vi "IMAQ-MWT (FPGA) without PA and Arduino Interface.vi"() -> ()   [LabVIEW 2015]
uses:
  <vilib>/eio/EIONode/EIONode.xnode
  <vilib>/rvi/eio/common/nirviEmuTemplateMethod_errors.vi
  <vilib>/Platform/TimedLoop/XDataNode/wakeup.ctl
  <vilib>/Platform/TimedLoop/XDataNode/XDNodeRunTimeDep.lvlib
  <vilib>/Platform/TimedLoop/XDataNode/nitl_modes.ctl
  <vilib>/Platform/TimedLoop/XDataNode/timing_clust.ctl
  <vilib>/Platform/TimedLoop/XDataNode/XDataNode.xnode
  Modules/Common/Controls (FPGA)/Pixel Bundle 40 Bytes.ctl
  <vilib>/rvi/DataTransferAndStorage/Container/XNode/niFpgaContainer.xnode
  <vilib>/rvi/FIFO/Fifo_Resource/nirvififoEmulationWrite.vi
  <vilib>/rvi/FIFO/Fifo_Resource/nirvififoEmulationRead.vi
  <vilib>/rvi/interface/RandomDataEmulation/nirviRandomDataFpgaReadWriteTemplate.vi
  Modules/CL Data to Pixels/8 Tap 8-Bit.vi
  Modules/CL Data to Pixels/10 Tap 8-Bit.vi
  Modules/Common/Controls (FPGA)/CL Configuration.ctl
  Modules/Common/Controls (FPGA)/CL Signal Mapping.ctl
  <vilib>/rvi/LocalResourceManager/LocalResourceManager.xnode
  <vilib>/rvi/DataTransferAndStorage/Container/Common/niFpgaContainerGetUniqueNameForEmu.vi
  <vilib>/rvi/DataTransferAndStorage/Container/Common/niFpgaContainerSetEmuInfo.vi
  <vilib>/rvi/eio/common/nirviEmuReportErrorAndStop.vi
  Modules/Common/Controls (FPGA)/Data to Arduino.ctl
  Modules/Common/Controls (FPGA)/Camera Tap Configuration.ctl
  Modules/Common/Controls (FPGA)/Run Mode.ctl
panel:
  in  "Baud Rate":u32=500000
  in  "N Spline Points":fxp<+,8,8>=31.0
  in  "Clock Cycles Limit":u32=10000
  in  "Pixel Intensity":cluster{"Low":u8, "High":u8}={"Low"=100, "High"=255}
  out "Frame Interval":u32=4294967295
  out "Frame #":u32
  out "DMA Timeout":bool
  in  "Mode":T1
  in  "Image Height":u16=3072
  in  "Image Width":u16=3072
  in  "Cancel Acq":bool
  in  "Acquire":bool
  out "Acq In Progress":bool
  in  "Tap Configuration":T2
  in  "Initialize":bool=TRUE
  out "Initialized":bool=TRUE
  # "IMAQ - MWT"
  # "Camera Link Configuration"
  # "Object Detection"
  # "Acquisition Settings"
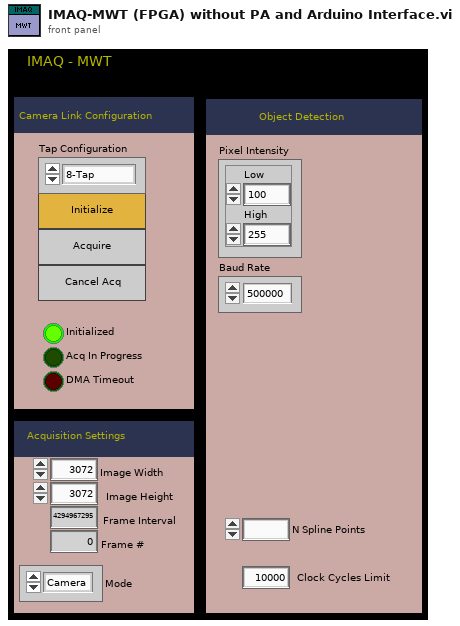
[diagram p1: front panel]
types:
  T1 = typedef "Run Mode.ctl" = enum16{"Camera", "Video (Raw)", "Video (DBDE)"}
  T2 = typedef "Camera Tap Configuration.ctl" = enum8{"8-Tap", "10-Tap"}
  T3 = typedef "CL Signal Mapping.ctl" = enum8{"Standard", "Basler 10-tap", "Vosskühler 10-tap"}
  T4 = typedef "CL Configuration.ctl" = enum8{"Base", "Medium", "Full"}
  T5 = typedef "XDNodeRunTimeDep.lvlib/timing_clust.ctl" = cluster{"Expected End [f-1]":u64, "Actual End [f-1]":u64, "Finished Late? [f-1]":bool, "Expected End [i-1]":u64, "Actual End [i-1]":u64, "Finished Late? [i-1]":bool, "Expected Start [i]":u64, "Actual Start [i]":u64, "Expected Start [f]":u64, "Actual Start [f]":u64, "Source Name":string, "Structure Name":string, "Period":i64, "Deadline":i64, "Offset":i64, "Start":i64, "Priority":i32, "Timeout":i32, "Mode":T6, "Wakeup Reason":T7, "Error":errorcluster, "Source Type":string, "Secondary Source Type":string, "Global End Time":u64, "Global Start Time":u64, "Frame Duration":u64, "Iteration Duration":u64, "Assigned CPU":i32, "I/O Scan Engine Mode":u32}
  T6 = typedef "XDNodeRunTimeDep.lvlib/nitl_modes.ctl" = enum32{"No Change", "Process missed periods, maintain original phase", "Discard missed periods, maintain original phase", "Process missed periods, ignore original phase", "Discard missed periods, ignore original phase"}
  T7 = typedef "XDNodeRunTimeDep.lvlib/wakeup.ctl" = enum32{"Normal", "Aborted", "Asynchronous wakeup", "Timing source error", "Timed loop error", "Timeout"}
  T8 = typedef "Pixel Bundle 40 Bytes.ctl" = cluster{"Pixel 1":u8, "Pixel 2":u8, "Pixel 3":u8, "Pixel 4":u8, "Pixel 5":u8, "Pixel 6":u8, "Pixel 7":u8, "Pixel 8":u8, "Pixel 9":u8, "Pixel 10":u8, "Pixel 11":u8, "Pixel 12":u8, "Pixel 13":u8, "Pixel 14":u8, "Pixel 15":u8, "Pixel 16":u8, "Pixel 17":u8, "Pixel 18":u8, "Pixel 19":u8, "Pixel 20":u8, "Pixel 21":u8, "Pixel 22":u8, "Pixel 23":u8, "Pixel 24":u8, "Pixel 25":u8, "Pixel 26":u8, "Pixel 27":u8, "Pixel 28":u8, "Pixel 29":u8, "Pixel 30":u8, "Pixel 31":u8, "Pixel 32":u8, "Pixel 33":u8, "Pixel 34":u8, "Pixel 35":u8, "Pixel 36":u8, "Pixel 37":u8, "Pixel 38":u8, "Pixel 39":u8, "Pixel 40":u8}
  T9 = cluster{"Enables Valid":bool, "Frame Valid":bool, "Line Valid":bool, "Data Valid":bool}
  T10 = cluster{"Pixel 0":u8, "Pixel 1":u8, "Pixel 2":u8, "Pixel 3":u8, "Pixel 4":u8, "Pixel 5":u8, "Pixel 6":u8, "Pixel 7":u8, "Pixel 8":u8, "Pixel 9":u8}
  T11 = cluster{"Pixel 0":u8, "Pixel 1":u8, "Pixel 2":u8, "Pixel 3":u8, "Pixel 4":u8, "Pixel 5":u8, "Pixel 6":u8, "Pixel 7":u8}
  T12 = cluster{"Pixel 1":u8, "Pixel 2":u8, "Pixel 3":u8, "Pixel 4":u8, "Pixel 5":u8, "Pixel 6":u8, "Pixel 7":u8, "Pixel 8":u8, "Pixel 9":u8, "Pixel 10":u8}
  T13 = typedef "Data to Arduino.ctl" = enum16{"SPINE Count", "SC 2", "SC 3", "SC 4", "SPINE Point", "SP 2", "SP 3", "SP 4", "End"}
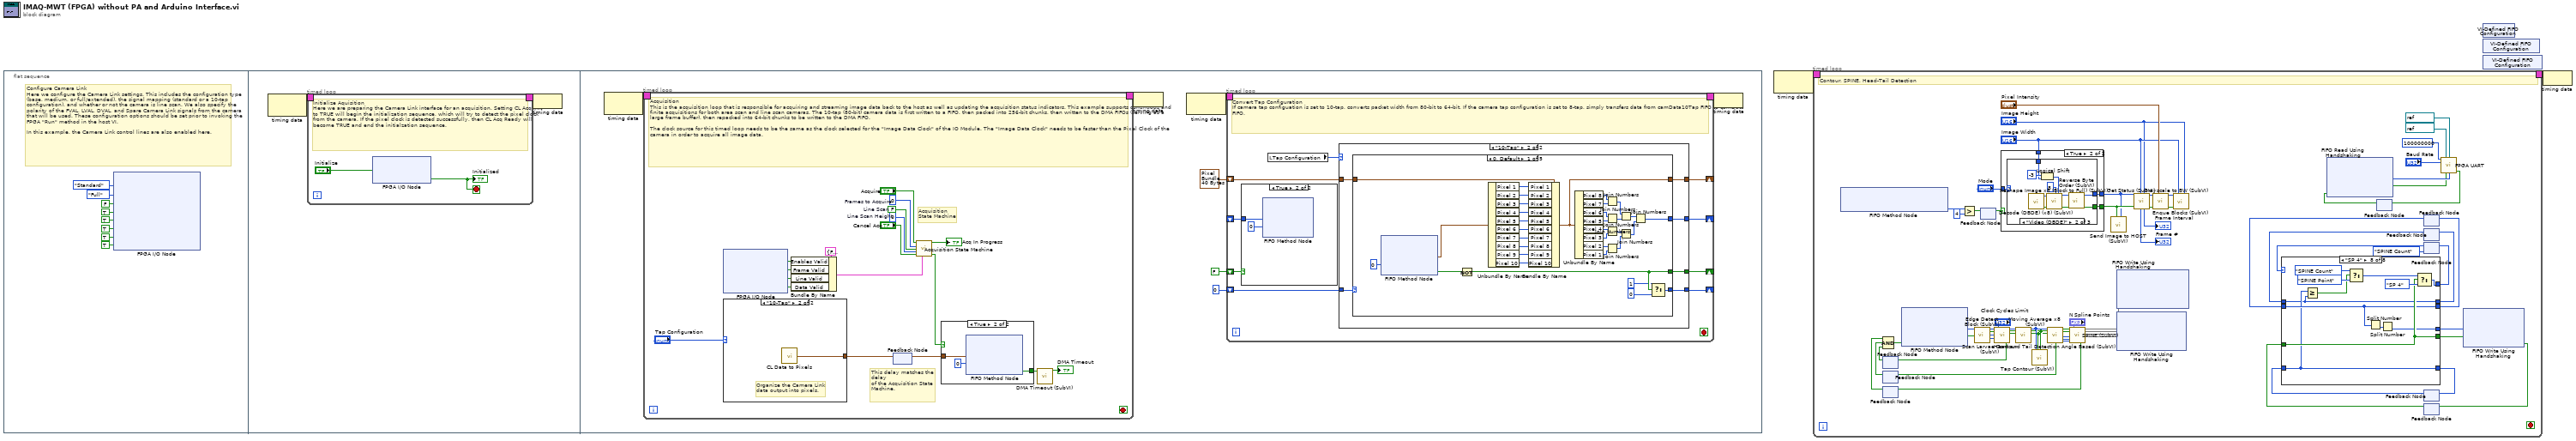
[diagram p0: block diagram]
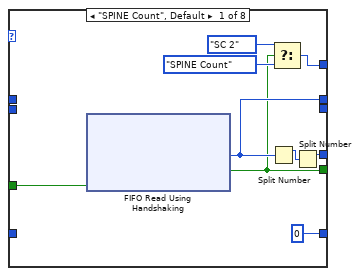
[diagram p2: hidden frame]
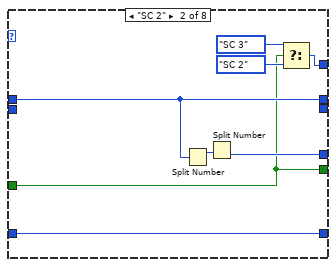
[diagram p3: hidden frame]
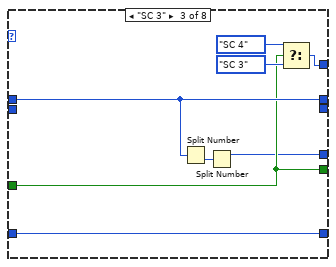
[diagram p4: hidden frame]
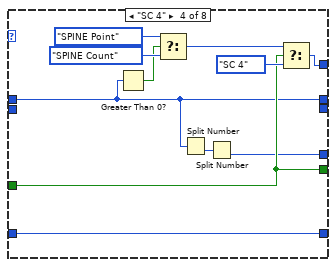
[diagram p5: hidden frame]
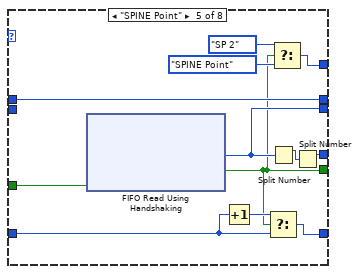
[diagram p6: hidden frame]
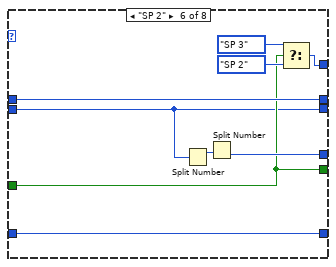
[diagram p7: hidden frame]
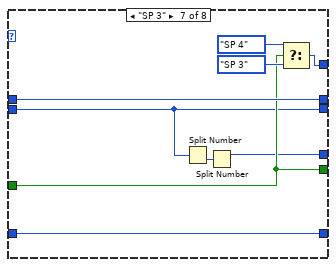
[diagram p8: hidden frame]
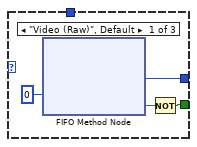
[diagram p10: hidden frame]
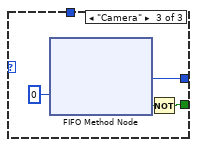
[diagram p11: hidden frame]
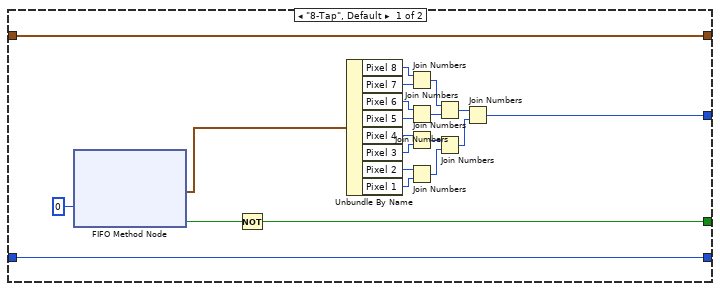
[diagram p13: hidden frame]
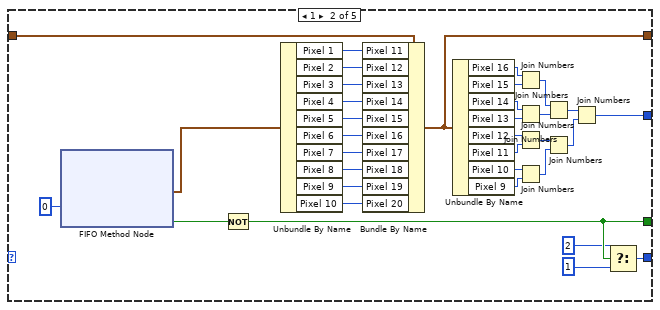
[diagram p14: hidden frame]
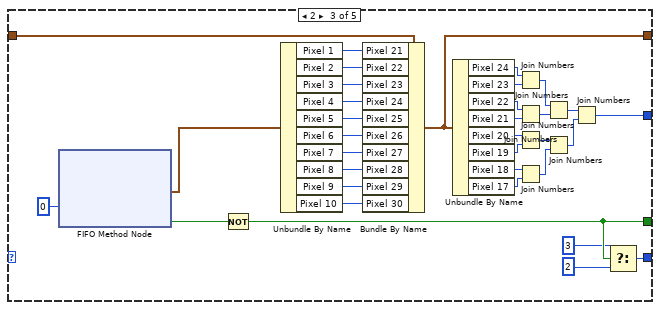
[diagram p15: hidden frame]
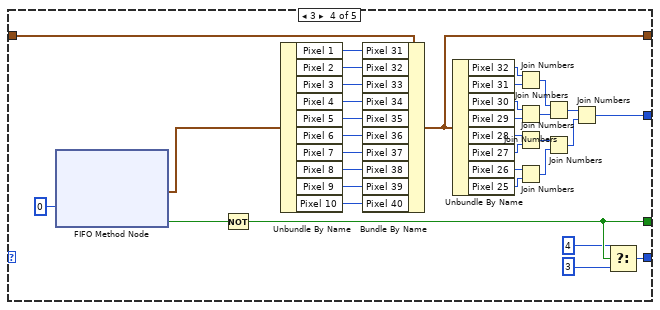
[diagram p16: hidden frame]
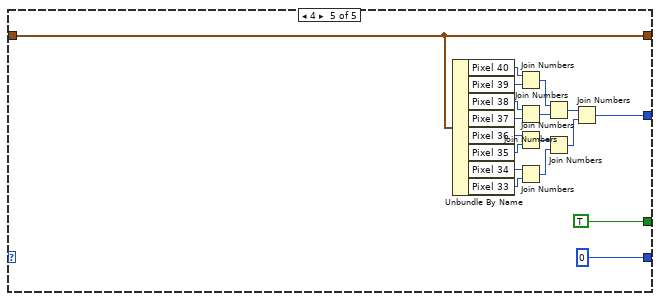
[diagram p17: hidden frame]
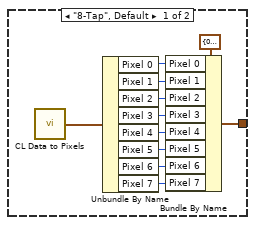
[diagram p18: hidden frame]
diagram:
  n1 = flat-sequence {
    frame #0 {
      # "Configure Camera Link\nHere we configure the Camera Link settings. This includes the configuration type (base, medium, or full/extended), the signal mapping (standard or a 10-tap configuration), and whether or not the camera is line scan. We also specify the polarity of the FVAL, LVAL, DVAL, and Spare Camera Link signals from the camera that will be used. These configuration options should be set prior to invoking the FPGA \"Run\" method in the host VI.\n\nIn this example, the Camera Link control lines are also enabled here."
      n2 = xnode "FPGA I/O Node"("CL Set Configuration"=CL_Signal_Mapping."Standard" ("Signal Mapping"), "CL Set Configuration"=CL_Configuration."Full" ("Configuration"), "CL Set Line Scan"=FALSE ("Line Scan"), "CL Set FVAL Active High"=TRUE ("FVAL Active High"), "CL Set LVAL Active High"=TRUE ("LVAL Active High"), "CL Set DVAL Active High"=TRUE ("DVAL Active High"), "CL Set Spare Active High"=TRUE ("Spare Active High"), "CL Control Enable"=TRUE ("IO Module\\CL Control Enable")) -> ()  [unwired: 8 in, 8 out]
    }
    frame #1 {
      n3 = node-c288() -> (w12:T5)  [unwired: 1 out]
      n4 = timed-loop {
        timing: w12 -> [_]
        timing-out: [_] -> w11
        stop <- w13 stop-if-true
        # "Initialize Aquisition\nHere we are preparing the Camera Link interface for an acquisition. Setting CL Acq Init to TRUE will begin the initialization sequence, which will try to detect the pixel clock from the camera. If the pixel clock is detected successfully, then CL Acq Ready will become TRUE and end the initialzation sequence."
        n5 = xnode "FPGA I/O Node"("CL Acq Init"="Initialize") -> ("CL Acq Ready"=w13:bool)  [unwired: 2 in, 2 out]
        "Initialized" <- w13
      }
      n6 = node-c288(w11) -> ()
    }
    frame #2 {
      n7 = node-c288() -> (w25:T5)  [unwired: 1 in]
      n8 = timed-loop {
        timing: w25 -> [_]
        timing-out: [_] -> w24
        stop <- _ stop-if-true
        w223 = FALSE  # Line Scan
        w224 = u32 0  # Line Scan Height
        w225 = u32 0  # Frames to Acquire
        # "This delay matches the delay\nof the Acquisition State Machine."
        # "Acquisition\nState Machine"
        # "Acquisition\nThis is the acquisition loop that is responsible for acquiring and streaming image data back to the host as well as updating the acquisition status indicators. This example supports continuous and finite acquisitions for both area scan and line scan cameras. The 10-tap (80-bit) camera data is first written to a FIFO, then packed into 256-bit chunks, then written to the DMA FIFOs (serving as a large frame buffer), then repacked into 64-bit chunks to be written to the DMA FIFO. \n\nThe clock source for this timed loop needs to be the same as the clock selected for the \"Image Data Clock\" of the IO Module. The \"Image Data Clock\" needs to be faster than the Pixel Clock of the camera in order to acquire all image data."
        n9 = xnode "FPGA I/O Node"() -> ("CL Output Valid"=w236:bool, "CL Frame Valid"=w235:bool, "CL Line Valid"=w234:bool, "CL Data Valid"=w232:bool)  [unwired: 4 in, 4 out]
        n10 = case shown="\"10-Tap\"" "Tap Configuration" {
          tunnel: [w240 w251] -> w228
          frame "8-Tap", Default {
            n11 = call-poly "CL Data to Pixels.vi"() -> ("Pixels"=w249:T11)  [unwired: 1 in]
            n12 = Unbundle By Name(w249) -> ("Pixel 0"=w248:u8, "Pixel 1"=w247:u8, "Pixel 2"=w246:u8, "Pixel 3"=w245:u8, "Pixel 4"=w244:u8, "Pixel 5"=w243:u8, "Pixel 6"=w242:u8, "Pixel 7"=w241:u8)
            n13 = Bundle By Name(cluster=T10 {"Pixel 0"=0, "Pixel 1"=0, "Pixel 2"=0, "Pixel 3"=0, "Pixel 4"=0, "Pixel 5"=0, "Pixel 6"=0, "Pixel 7"=0, "Pixel 8"=0, "Pixel 9"=0} ("Pixels"), "Pixel 0"=w248, "Pixel 1"=w247, "Pixel 2"=w246, "Pixel 3"=w245, "Pixel 4"=w244, "Pixel 5"=w243, "Pixel 6"=w242, "Pixel 7"=w241) -> (w240:T10)
          }
          frame "10-Tap" {
            # "Organize the Camera Link\ndata output into pixels."
            n14 = call-poly "CL Data to Pixels.vi"() -> ("Pixels"=w251:T10)  [unwired: 1 in]
          }
        }
        n15 = Bundle By Name(cluster=T9 {"Enables Valid"=FALSE, "Frame Valid"=FALSE, "Line Valid"=FALSE, "Data Valid"=FALSE} ("Enables"), "Enables Valid"=w236, "Frame Valid"=w235, "Line Valid"=w234, "Data Valid"=w232) -> (w233:T9)
        n16 = feedback-in #1(w228) -> ()
        n17 = feedback #1() -> (w229:T10)  [unwired: 1 in]
        n18 = call "Acquisition State Machine.vi"("Acquire"="Acquire", "Frames to Acquire"=w225, "Line Scan"=w223, "Line Scan Height"=w224, "Cancel Acq"="Cancel Acq", "Enables"=w233) -> ("Acq In Progress"=→"Acq In Progress":bool, "Capture Cycle"=w230:bool)  [unwired: 4 in, 4 out]
        n19 = case shown="True" w230 {
          tunnel: [_ w252] -> w226
          tunnel: w229 -> [_ w253]
          frame False {
          }
          frame True {
            n20 = xnode ("FIFO Method Node")("Element"=w253, "Timeout"=0) -> ("Timed Out?"=w252:bool)  [unwired: 1 in, 1 out]
          }
        }
        n21 = call "DMA Timeout (SubVI).vi"("Timeout"=w226) -> ("DMA Timeout"=→"DMA Timeout":bool)  [unwired: 10 in]
      }
      n22 = node-c288(w24) -> ()
      n23 = node-c288() -> (w23:T5)  [unwired: 1 in]
      n24 = timed-loop {
        timing: w23 -> [_]
        timing-out: [_] -> w22
        shift-right: [w32] -> _
        shift-left: u8 0 ("Timeout") -> [w33]
        shift-right: [w30] -> _
        shift-left: T8 {"Pixel 1"=0, "Pixel 2"=0, "Pixel 3"=0, "Pixel 4"=0, "Pixel 5"=0, "Pixel 6"=0, "Pixel 7"=0, "Pixel 8"=0, "Pixel 9"=0, "Pixel 10"=0, "Pixel 11"=0, "Pixel 12"=0, "Pixel 13"=0, "Pixel 14"=0, "Pixel 15"=0, "Pixel 16"=0, "Pixel 17"=0, "Pixel 18"=0, "Pixel 19"=0, "Pixel 20"=0, "Pixel 21"=0, "Pixel 22"=0, "Pixel 23"=0, "Pixel 24"=0, "Pixel 25"=0, "Pixel 26"=0, "Pixel 27"=0, "Pixel 28"=0, "Pixel 29"=0, "Pixel 30"=0, "Pixel 31"=0, "Pixel 32"=0, "Pixel 33"=0, "Pixel 34"=0, "Pixel 35"=0, "Pixel 36"=0, "Pixel 37"=0, "Pixel 38"=0, "Pixel 39"=0, "Pixel 40"=0} ("Data In") -> [w31]
        shift-right: [w29] -> _
        shift-left: _ -> [w26]
        shift-right: [w28] -> _
        shift-left: FALSE -> [w27]
        stop <- _ stop-if-true
        # "Convert Tap Configuration\nIf camera tap configuation is set to 10-tap, converts packet width from 80-bit to 64-bit. If the camera tap configuration is set to 8-tap, simply transfers data from camData10Tap FIFO to camData FIFO."
        n25 = case shown="True" w27 {
          tunnel: w26 -> [_ w36]
          frame False {
          }
          frame True {
            n26 = xnode ("FIFO Method Node")("Element"=w36, "Timeout"=0) -> ()  [unwired: 1 in, 2 out]
          }
        }
        n27 = local read "Tap Configuration"() -> (w34:T2)
        n28 = case shown="\"10-Tap\"" w34 {
          tunnel: [w43 w62] -> w28
          tunnel: [w42 w61] -> w29
          tunnel: w33 -> [w41 w63]
          tunnel: [w41 w60] -> w32
          tunnel: w31 -> [w40 w59]
          tunnel: [w40 w58] -> w30
          frame "8-Tap", Default {
            n29 = xnode ("FIFO Method Node")("Timeout"=0) -> ("Element"=w39:T12, "Timed Out?"=w38:bool)  [unwired: 1 in, 1 out]
            n30 = Not(x=w38) -> (.not. x?=w43:bool)
            n31 = Unbundle By Name(w39) -> ("Pixel 8"=w57:u8, "Pixel 7"=w56:u8, "Pixel 6"=w55:u8, "Pixel 5"=w54:u8, "Pixel 4"=w52:u8, "Pixel 3"=w53:u8, "Pixel 2"=w50:u8, "Pixel 1"=w51:u8)
            n32 = Join Numbers(hi=w57, lo=w56) -> ((hi.lo)=w48:u16)
            n33 = Join Numbers(hi=w55, lo=w54) -> ((hi.lo)=w49:u16)
            n34 = Join Numbers(hi=w52, lo=w53) -> ((hi.lo)=w47:u16)
            n35 = Join Numbers(hi=w50, lo=w51) -> ((hi.lo)=w46:u16)
            n36 = Join Numbers(hi=w48, lo=w49) -> ((hi.lo)=w45:u32)
            n37 = Join Numbers(hi=w47, lo=w46) -> ((hi.lo)=w44:u32)
            n38 = Join Numbers(hi=w45, lo=w44) -> ((hi.lo)=w42:u64)
          }
          frame "10-Tap" {
            n39 = case shown="0, Default" w63 {
              tunnel: [w81 w115 w149 w183 TRUE] -> w62
              tunnel: [w83 w117 w151 w185 w203] -> w61
              tunnel: [w82 w116 w150 w184 u8 0 ("Timeout")] -> w60
              tunnel: w59 -> [w78 w112 w146 w180 w202]
              tunnel: [w77 w111 w145 w179 w202] -> w58
              frame 0, Default {
                n40 = xnode ("FIFO Method Node")("Timeout"=0) -> ("Element"=w65:T12, "Timed Out?"=w66:bool)  [unwired: 1 in, 1 out]
                n41 = Not(x=w66) -> (.not. x?=w81:bool)
                n42 = Unbundle By Name(w65) -> ("Pixel 1"=w76:u8, "Pixel 2"=w75:u8, "Pixel 3"=w74:u8, "Pixel 4"=w73:u8, "Pixel 5"=w72:u8, "Pixel 6"=w71:u8, "Pixel 7"=w70:u8, "Pixel 8"=w69:u8, "Pixel 9"=w68:u8, "Pixel 10"=w67:u8)
                n43 = Bundle By Name(cluster=w78, "Pixel 1"=w76, "Pixel 2"=w75, "Pixel 3"=w74, "Pixel 4"=w73, "Pixel 5"=w72, "Pixel 6"=w71, "Pixel 7"=w70, "Pixel 8"=w69, "Pixel 9"=w68, "Pixel 10"=w67) -> (w77:T8)
                n44 = Unbundle By Name(w77) -> ("Pixel 8"=w97:u8, "Pixel 7"=w96:u8, "Pixel 6"=w95:u8, "Pixel 5"=w94:u8, "Pixel 4"=w92:u8, "Pixel 3"=w93:u8, "Pixel 2"=w90:u8, "Pixel 1"=w91:u8)
                n45 = Join Numbers(hi=w97, lo=w96) -> ((hi.lo)=w88:u16)
                n46 = Join Numbers(hi=w95, lo=w94) -> ((hi.lo)=w89:u16)
                n47 = Join Numbers(hi=w92, lo=w93) -> ((hi.lo)=w87:u16)
                n48 = Join Numbers(hi=w90, lo=w91) -> ((hi.lo)=w86:u16)
                n49 = Join Numbers(hi=w88, lo=w89) -> ((hi.lo)=w85:u32)
                n50 = Join Numbers(hi=w87, lo=w86) -> ((hi.lo)=w84:u32)
                n51 = Join Numbers(hi=w85, lo=w84) -> ((hi.lo)=w83:u64)
                n52 = Select(t=u8 1 ("Timeout"), s=w81, f=u8 0 ("Timeout")) -> (s? t:f=w82:u8)
              }
              frame 1 {
                n53 = xnode ("FIFO Method Node")("Timeout"=0) -> ("Element"=w100:T12, "Timed Out?"=w99:bool)  [unwired: 1 in, 1 out]
                n54 = Not(x=w99) -> (.not. x?=w115:bool)
                n55 = Unbundle By Name(w100) -> ("Pixel 1"=w110:u8, "Pixel 2"=w109:u8, "Pixel 3"=w108:u8, "Pixel 4"=w107:u8, "Pixel 5"=w106:u8, "Pixel 6"=w105:u8, "Pixel 7"=w104:u8, "Pixel 8"=w103:u8, "Pixel 9"=w102:u8, "Pixel 10"=w101:u8)
                n56 = Bundle By Name(cluster=w112, "Pixel 11"=w110, "Pixel 12"=w109, "Pixel 13"=w108, "Pixel 14"=w107, "Pixel 15"=w106, "Pixel 16"=w105, "Pixel 17"=w104, "Pixel 18"=w103, "Pixel 19"=w102, "Pixel 20"=w101) -> (w111:T8)
                n57 = Unbundle By Name(w111) -> ("Pixel 16"=w131:u8, "Pixel 15"=w130:u8, "Pixel 14"=w129:u8, "Pixel 13"=w128:u8, "Pixel 12"=w126:u8, "Pixel 11"=w127:u8, "Pixel 10"=w124:u8, "Pixel 9"=w125:u8)
                n58 = Join Numbers(hi=w131, lo=w130) -> ((hi.lo)=w122:u16)
                n59 = Join Numbers(hi=w129, lo=w128) -> ((hi.lo)=w123:u16)
                n60 = Join Numbers(hi=w126, lo=w127) -> ((hi.lo)=w121:u16)
                n61 = Join Numbers(hi=w124, lo=w125) -> ((hi.lo)=w120:u16)
                n62 = Join Numbers(hi=w122, lo=w123) -> ((hi.lo)=w119:u32)
                n63 = Join Numbers(hi=w121, lo=w120) -> ((hi.lo)=w118:u32)
                n64 = Join Numbers(hi=w119, lo=w118) -> ((hi.lo)=w117:u64)
                n65 = Select(t=u8 2 ("Timeout"), s=w115, f=u8 1 ("Timeout")) -> (s? t:f=w116:u8)
              }
              frame 2 {
                n66 = xnode ("FIFO Method Node")("Timeout"=0) -> ("Element"=w133:T12, "Timed Out?"=w134:bool)  [unwired: 1 in, 1 out]
                n67 = Not(x=w134) -> (.not. x?=w149:bool)
                n68 = Unbundle By Name(w133) -> ("Pixel 1"=w144:u8, "Pixel 2"=w143:u8, "Pixel 3"=w142:u8, "Pixel 4"=w141:u8, "Pixel 5"=w140:u8, "Pixel 6"=w139:u8, "Pixel 7"=w138:u8, "Pixel 8"=w137:u8, "Pixel 9"=w136:u8, "Pixel 10"=w135:u8)
                n69 = Bundle By Name(cluster=w146, "Pixel 21"=w144, "Pixel 22"=w143, "Pixel 23"=w142, "Pixel 24"=w141, "Pixel 25"=w140, "Pixel 26"=w139, "Pixel 27"=w138, "Pixel 28"=w137, "Pixel 29"=w136, "Pixel 30"=w135) -> (w145:T8)
                n70 = Unbundle By Name(w145) -> ("Pixel 24"=w165:u8, "Pixel 23"=w164:u8, "Pixel 22"=w163:u8, "Pixel 21"=w162:u8, "Pixel 20"=w160:u8, "Pixel 19"=w161:u8, "Pixel 18"=w158:u8, "Pixel 17"=w159:u8)
                n71 = Join Numbers(hi=w165, lo=w164) -> ((hi.lo)=w156:u16)
                n72 = Join Numbers(hi=w163, lo=w162) -> ((hi.lo)=w157:u16)
                n73 = Join Numbers(hi=w160, lo=w161) -> ((hi.lo)=w155:u16)
                n74 = Join Numbers(hi=w158, lo=w159) -> ((hi.lo)=w154:u16)
                n75 = Join Numbers(hi=w156, lo=w157) -> ((hi.lo)=w153:u32)
                n76 = Join Numbers(hi=w155, lo=w154) -> ((hi.lo)=w152:u32)
                n77 = Join Numbers(hi=w153, lo=w152) -> ((hi.lo)=w151:u64)
                n78 = Select(t=u8 3 ("Timeout"), s=w149, f=u8 2 ("Timeout")) -> (s? t:f=w150:u8)
              }
              frame 3 {
                n79 = xnode ("FIFO Method Node")("Timeout"=0) -> ("Element"=w167:T12, "Timed Out?"=w168:bool)  [unwired: 1 in, 1 out]
                n80 = Not(x=w168) -> (.not. x?=w183:bool)
                n81 = Unbundle By Name(w167) -> ("Pixel 1"=w178:u8, "Pixel 2"=w177:u8, "Pixel 3"=w176:u8, "Pixel 4"=w175:u8, "Pixel 5"=w174:u8, "Pixel 6"=w173:u8, "Pixel 7"=w172:u8, "Pixel 8"=w171:u8, "Pixel 9"=w170:u8, "Pixel 10"=w169:u8)
                n82 = Bundle By Name(cluster=w180, "Pixel 31"=w178, "Pixel 32"=w177, "Pixel 33"=w176, "Pixel 34"=w175, "Pixel 35"=w174, "Pixel 36"=w173, "Pixel 37"=w172, "Pixel 38"=w171, "Pixel 39"=w170, "Pixel 40"=w169) -> (w179:T8)
                n83 = Unbundle By Name(w179) -> ("Pixel 32"=w199:u8, "Pixel 31"=w198:u8, "Pixel 30"=w197:u8, "Pixel 29"=w196:u8, "Pixel 28"=w194:u8, "Pixel 27"=w195:u8, "Pixel 26"=w192:u8, "Pixel 25"=w193:u8)
                n84 = Join Numbers(hi=w199, lo=w198) -> ((hi.lo)=w190:u16)
                n85 = Join Numbers(hi=w197, lo=w196) -> ((hi.lo)=w191:u16)
                n86 = Join Numbers(hi=w194, lo=w195) -> ((hi.lo)=w189:u16)
                n87 = Join Numbers(hi=w192, lo=w193) -> ((hi.lo)=w188:u16)
                n88 = Join Numbers(hi=w190, lo=w191) -> ((hi.lo)=w187:u32)
                n89 = Join Numbers(hi=w189, lo=w188) -> ((hi.lo)=w186:u32)
                n90 = Join Numbers(hi=w187, lo=w186) -> ((hi.lo)=w185:u64)
                n91 = Select(t=u8 4 ("Timeout"), s=w183, f=u8 3 ("Timeout")) -> (s? t:f=w184:u8)
              }
              frame 4 {
                n92 = Unbundle By Name(w202) -> ("Pixel 40"=w217:u8, "Pixel 39"=w216:u8, "Pixel 38"=w215:u8, "Pixel 37"=w214:u8, "Pixel 36"=w212:u8, "Pixel 35"=w213:u8, "Pixel 34"=w210:u8, "Pixel 33"=w211:u8)
                n93 = Join Numbers(hi=w217, lo=w216) -> ((hi.lo)=w208:u16)
                n94 = Join Numbers(hi=w215, lo=w214) -> ((hi.lo)=w209:u16)
                n95 = Join Numbers(hi=w212, lo=w213) -> ((hi.lo)=w207:u16)
                n96 = Join Numbers(hi=w210, lo=w211) -> ((hi.lo)=w206:u16)
                n97 = Join Numbers(hi=w208, lo=w209) -> ((hi.lo)=w205:u32)
                n98 = Join Numbers(hi=w207, lo=w206) -> ((hi.lo)=w204:u32)
                n99 = Join Numbers(hi=w205, lo=w204) -> ((hi.lo)=w203:u64)
              }
            }
          }
        }
      }
      n100 = node-c288(w22) -> ()
    }
  }
  n101 = node-c288() -> (w2:T5)  [unwired: 1 in]
  n102 = timed-loop {
    timing: w2 -> [_]
    timing-out: [_] -> w1
    stop <- _ stop-if-true
    # "Contour, SPINE, Head-Tail Detection"
    n103 = xnode ("FIFO Method Node")() -> ("Number of Elements to Write"=w307:u32)  [unwired: 1 in, 1 out]
    n104 = feedback #2() -> (w314:bool)  [unwired: 1 in]
    n105 = feedback #3() -> (w315:bool)  [unwired: 1 in]
    n106 = feedback #4() -> (w313:bool)  [unwired: 1 in]
    n107 = Compound Arithmetic op=AND(w313, w315, w314) -> (w306:bool)
    n108 = xnode ("FIFO Method Node")("Ready for Output"=w306) -> ("Element"=w305:u8, "Output Valid"=w304:bool)  [unwired: 1 in, 1 out]
    n109 = Greater?(x=w307, y=u32 4) -> (0:w311:bool)
    n110 = call "Edge Detect Block (SubVI).vi"("Data In"=w305, "In Valid?"=w304) -> ("Data Out"=w303:u8, "Out Valid?"=w302:bool, "X Start"=w316:u16, "Y Start"=w317:u16)  [unwired: 10 in]
    n111 = feedback-in #5(w311) -> ()
    n112 = feedback #5() -> (w310:bool)  [unwired: 1 in]
    n113 = call "Scan Larvae Contour (SubVI).vi"("Data In"=w303, "Input Valid?"=w302, "X Start"=w316, "Y Start"=w317, "Max. Scan Cycles"="Clock Cycles Limit") -> ("Ready for Input?"=w288:bool, "Boundary Point XY"=w294:u32, "Boundary Valid?"=w293:bool, "Scan End?"=w292:bool)  [unwired: 10 in, 1 out]
    n114 = feedback-in #2(w288) -> ()
    n115 = case shown="True" w310 {
      tunnel: "Mode" -> [_ w407]
      tunnel: "Image Width" -> [_ w406]
      tunnel: [_ w405] -> w284
      tunnel: [_ w404] -> w285
      frame False {
      }
      frame True {
        n116 = case shown="\"Video (DBDE)\"" w407 {
          tunnel: [w411 w416 w424] -> w404
          tunnel: [w410 w417 w423] -> w405
          tunnel: w406 -> [_ w414 _]
          frame "Video (Raw)", Default {
            n117 = xnode ("FIFO Method Node")("Timeout"=0) -> ("Element"=w410:u64, "Timed Out?"=w409:bool)  [unwired: 1 in, 1 out]
            n118 = Not(x=w409) -> (.not. x?=w411:bool)
          }
          frame "Video (DBDE)" {
            n119 = call "Decode (DBDE) (x8) (SubVI).vi"() -> ("Output Valid"=w419:bool, "Data Out"=w418:u64)  [unwired: 10 in]
            n120 = Logical Shift(y=i16 -3, x=w414) -> (x << y=w413:u16)
            n121 = call "Reshape Image x8 (Block to Full) (SubVI).vi"("Pixel Data In"=w418, "Pixel In Valid?"=w419, "Block Size"=u16 8, "Image Width (/8)"=w413) -> ("Pixel Data Out"=w420:u64, "Pixel Out Valid?"=w416:bool)  [unwired: 14 in]
            n122 = call "Reverse Byte Order (SubVI).vi"("Data In"=w420) -> ("Data Out"=w417:u64)  [unwired: 10 in]
          }
          frame "Camera" {
            n123 = xnode ("FIFO Method Node")("Timeout"=0) -> ("Element"=w423:u64, "Timed Out?"=w422:bool)  [unwired: 1 in, 1 out]
            n124 = Not(x=w422) -> (.not. x?=w424:bool)
          }
        }
      }
    }
    n125 = call "Moving Average x8 (SubVI).vi"("Point In"=w294, "Boundary Valid? In"=w293, "Scan End? In"=w292) -> ("Point Out"=w291:u32, "Boundary Valid? out"=w290:bool, "Scan End? Out"=w289:bool)  [unwired: 14 in]
    n126 = call "Tap Contour (SubVI).vi"("Contour XY"=w291, "Complete?"=w289, "Input Valid?"=w290) -> ()  [unwired: 17 in]
    n127 = call "Head and Tail Detection Angle Based (SubVI).vi"("Boundary Point XY"=w291, "Bondary Valid?"=w290, "Scan End?"=w289) -> ("Ready for Input?"=w287:bool, "Output Valid?"=w296:bool, "Skip Contour Analysis"=w297:bool, "V1 (ID)"=w298:u16, "V2 (ID)"=w299:u16, "N Points"=w300:u16)  [unwired: 9 in, 2 out]
    n128 = feedback-in #3(w287) -> ()
    n129 = call "SPINE (SubVI).vi"("Input Valid?"=w296, "Skip SPLINE?"=w297, "V1 (ID)"=w298, "V2 (ID)"=w299, "N Points"=w300, "N Spline Points"="N Spline Points") -> ("Ready for Input?"=w286:bool, 14:w283, 15:w282, 16:w281, 17:w280)  [unwired: 9 in]
    n130 = feedback-in #4(w286) -> ()
    n131 = call "Send Image to HOST (SubVI).vi"("Pixel Data"=w284, "Input Valid"=w285) -> ()  [unwired: 10 in]
    n132 = xnode ("FIFO Write Using Handshaking")("Element"=w283, "Input Valid"=w282) -> ()  [unwired: 1 in, 2 out]
    n133 = xnode ("FIFO Write Using Handshaking")("Element"=w281, "Input Valid"=w280) -> ()  [unwired: 1 in, 2 out]
    n134 = call "Get Status (SubVI).vi"("Image Height"="Image Height", "Image Width"="Image Width", "Input Valid?"=w285, "Pixel In"=w284) -> ("Pixel Valid?"=w323:bool, "Pixel Out"=w322:u64, "Frame Interval"=→"Frame Interval":u32, "Frame #"=→"Frame #":u32)  [unwired: 4 in]
    n135 = call "Grayscale to BW (SubVI).vi"("Threshold Range"="Pixel Intensity", "Input Valid"=w323, "Data In"=w322) -> ("Output Valid"=w308:bool, "Data Out"=w309:u64)  [unwired: 7 in]
    n136 = call "Enque Blocks (SubVI).vi"("Pixels In"=w309, "Image Width"="Image Width", "Image Height"="Image Height", "Input Valid?"=w308) -> ()  [unwired: 11 in, 1 out]
    n137 = feedback #6() -> (w266:bool)  [unwired: 1 in]
    n138 = xnode ("FIFO Read Using Handshaking")("Ready for Output"=w266) -> ("Element"=w264:u8, "Output Valid"=w263:bool)  [unwired: 1 in, 1 out]
    n139 = feedback #7() -> (w279:u32)  [unwired: 1 in]
    n140 = feedback #8() -> (w267:bool)  [unwired: 1 in]
    n141 = feedback #9() -> (w277:u32)  [unwired: 1 in]
    n142 = feedback #10() -> (w271:u32)  [unwired: 1 in]
    n143 = feedback #11(Data_to_Arduino."SPINE Count") -> (w274:T13)
    n144 = case shown="\"SP 4\"" w274 {
      tunnel: [w332 w338 w348 w360 w371 w378 w389 w402] -> w275
      tunnel: w267 -> [w333 w336 w346 w359 w372 w376 w387 w401]
      tunnel: [w330 w341 w350 w354 w367 w381 w391 w395] -> w272
      tunnel: w271 -> [_ w341 w350 w354 w367 w381 w391 w395]
      tunnel: [w328 w340 w345 w357 w368 w380 w383 w392] -> w270
      tunnel: [w327 w336 w346 w359 w362 w376 w387 w401] -> w269
      tunnel: [_ _ _ _ w366 w375 w386 w400] -> w276
      tunnel: w277 -> [_ _ _ _ _ w375 w386 w400]
      tunnel: [u32 0 ("Element") w335 w343 w351 w365 w374 w385 w396] -> w278
      tunnel: w279 -> [_ w335 w343 w351 w363 w374 w385 w396]
      frame "SPINE Count", Default {
        n145 = xnode ("FIFO Read Using Handshaking")("Ready for Output"=w333) -> ("Element"=w330:u32, "Output Valid"=w327:bool)  [unwired: 1 in, 1 out]
        n146 = Split Number(x=w330) -> (hi(x)=w329:u16)  [unwired: 1 out]
        n147 = Select(t=Data_to_Arduino."SC 2", s=w327, f=Data_to_Arduino."SPINE Count") -> (s? t:f=w332:T13)
        n148 = Split Number(x=w329) -> (hi(x)=w328:u8)  [unwired: 1 out]
      }
      frame "SC 2" {
        n149 = Split Number(x=w341) -> (hi(x)=w342:u16)  [unwired: 1 out]
        n150 = Split Number(x=w342) -> (lo(x)=w340:u8)  [unwired: 1 out]
        n151 = Select(t=Data_to_Arduino."SC 3", s=w336, f=Data_to_Arduino."SC 2") -> (s? t:f=w338:T13)
      }
      frame "SC 3" {
        n152 = Split Number(x=w350) -> (lo(x)=w344:u16)  [unwired: 1 out]
        n153 = Split Number(x=w344) -> (hi(x)=w345:u8)  [unwired: 1 out]
        n154 = Select(t=Data_to_Arduino."SC 4", s=w346, f=Data_to_Arduino."SC 3") -> (s? t:f=w348:T13)
      }
      frame "SC 4" {
        n155 = Greater Than 0?(x=w354) -> (x > 0?=w352:bool)
        n156 = Select(t=Data_to_Arduino."SPINE Point", s=w352, f=Data_to_Arduino."SPINE Count") -> (s? t:f=w353:T13)
        n157 = Split Number(x=w354) -> (lo(x)=w358:u16)  [unwired: 1 out]
        n158 = Split Number(x=w358) -> (lo(x)=w357:u8)  [unwired: 1 out]
        n159 = Select(t=w353, s=w359, f=Data_to_Arduino."SC 4") -> (s? t:f=w360:T13)
      }
      frame "SPINE Point" {
        n160 = xnode ("FIFO Read Using Handshaking")("Ready for Output"=w372) -> ("Element"=w366:u32, "Output Valid"=w362:bool)  [unwired: 1 in, 1 out]
        n161 = Increment(x=w363) -> (x+1=w364:u32)
        n162 = Select(t=w364, s=w362, f=w363) -> (s? t:f=w365:u32)
        n163 = Split Number(x=w366) -> (hi(x)=w369:u16)  [unwired: 1 out]
        n164 = Select(t=Data_to_Arduino."SP 2", s=w362, f=Data_to_Arduino."SPINE Point") -> (s? t:f=w371:T13)
        n165 = Split Number(x=w369) -> (hi(x)=w368:u8)  [unwired: 1 out]
      }
      frame "SP 2" {
        n166 = Split Number(x=w375) -> (hi(x)=w382:u16)  [unwired: 1 out]
        n167 = Split Number(x=w382) -> (lo(x)=w380:u8)  [unwired: 1 out]
        n168 = Select(t=Data_to_Arduino."SP 3", s=w376, f=Data_to_Arduino."SP 2") -> (s? t:f=w378:T13)
      }
      frame "SP 3" {
        n169 = Split Number(x=w386) -> (lo(x)=w384:u16)  [unwired: 1 out]
        n170 = Split Number(x=w384) -> (hi(x)=w383:u8)  [unwired: 1 out]
        n171 = Select(t=Data_to_Arduino."SP 4", s=w387, f=Data_to_Arduino."SP 3") -> (s? t:f=w389:T13)
      }
      frame "SP 4" {
        n172 = Greater Or Equal?(x=w396, y=w395) -> (x >= y?=w394:bool)
        n173 = Select(t=Data_to_Arduino."SPINE Count", s=w394, f=Data_to_Arduino."SPINE Point") -> (s? t:f=w397:T13)
        n174 = Split Number(x=w400) -> (lo(x)=w399:u16)  [unwired: 1 out]
        n175 = Split Number(x=w399) -> (lo(x)=w392:u8)  [unwired: 1 out]
        n176 = Select(t=w397, s=w401, f=Data_to_Arduino."SP 4") -> (s? t:f=w402:T13)
      }
    }
    n177 = feedback-in #7(w278) -> ()
    n178 = feedback-in #9(w276) -> ()
    n179 = feedback-in #10(w272) -> ()
    n180 = feedback-in #11(w275) -> ()
    n181 = call "FPGA UART.vi"("Clock Frequency"=u32 100000000, "Tx IO"=refnum<k21> "TTL 1", "Rx IO"=refnum<k21> "TTL 2", "Baud Rate"="Baud Rate", "Input Valid?"=w263, "Tx Data"=w264) -> ("Ready for Input?"=w265:bool)  [unwired: 7 in, 2 out]
    n182 = feedback-in #6(w265) -> ()
    n183 = xnode ("FIFO Write Using Handshaking")("Element"=w270, "Input Valid"=w269) -> ("Ready for Input"=w268:bool)  [unwired: 1 in, 1 out]
    n184 = feedback-in #8(w268) -> ()
  }
  n185 = xnode "VI-Defined FIFO Configuration"() -> ()  [unwired: 1 out]
  n186 = xnode "VI-Defined FIFO Configuration"() -> ()  [unwired: 1 out]
  n187 = xnode "VI-Defined FIFO Configuration"() -> ()  [unwired: 1 out]
  n188 = node-c288(w1) -> ()
